vi "timestamp to timeval.vi"(11 "seconds since 1Jan1904":timestamp) -> (3 "timeval":T1)   [LabVIEW 2020, in "libpcaplv.lvlib"]
uses:
  libpcaplv.lvlib
  _typedefs/timeval_type_x64.ctl
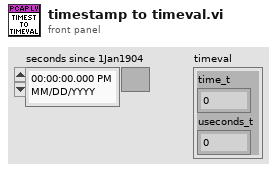
[diagram p1: front panel]
types:
  T1 = typedef "libpcaplv.lvlib/timeval_type_x64.ctl" = cluster{"time_t":u64, "useconds_t":u64}
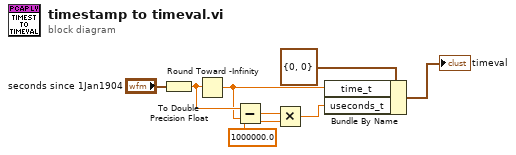
[diagram p0: block diagram]
diagram:
  n1 = To Double Precision Float(number="seconds since 1Jan1904") -> (double precision float=w3:dbl)
  n2 = Round Toward -Infinity(1:w3) -> (0:w1:dbl)
  n3 = Subtract(x=w3, y=w1) -> (x-y=w4:dbl)
  n4 = Multiply(x=w4, y=1000000.0) -> (x*y=w8:dbl)
  n5 = Bundle By Name(cluster=T1 {"time_t"=0, "useconds_t"=0} ("timeval"), "time_t"=w1, "useconds_t"=w8) -> (→"timeval":T1)
